vi "Biostinger GUI.vi"() -> ()   [LabVIEW 2014]
uses:
  Controls/State_Enum.ctl
  <vilib>/Utility/file.llb/Write To Spreadsheet File (DBL).vi
panel:
  in  "Clear":bool
  in  "Retraction (um)":dbl
  in  "Penetration (um)":dbl
  out "Waveform Graph":dbl[](graph)
  in  "Zero":bool
  out "XY Graph":cluster{dbl, dbl}[](graph)
  in  "Start Experiment":bool
  in  "Save File":path
  in  "Duration (ms)":u16
  in  "End Voltage (mV)":i16
  in  "Pulse Voltage (mV)":i16
  in  "Current Voltage (mV)":i16
  in  "Command":T1(ring)=enum."Set Statuses"
  in  "Status Value":u16 format="%04x"
  in  "Status Number":u8=61
  in  "Send Command":bool
  out "(hi.lo)":u32[](array[numeric]) format="%8x"
  out "Read Data 4":i32[](array[numeric]) format="%02d"
  in  "Set Parameters":bool
  in  "Start":bool
  in  "Stop":bool
  out "Read Data":u8[](array[numeric]) format="%02x"
  out "Status":string
  out "error out":errorcluster
  in  "error in (no error)":errorcluster
  # "Set Parameters"
  # "Record Data"
  # "Start Experiment"
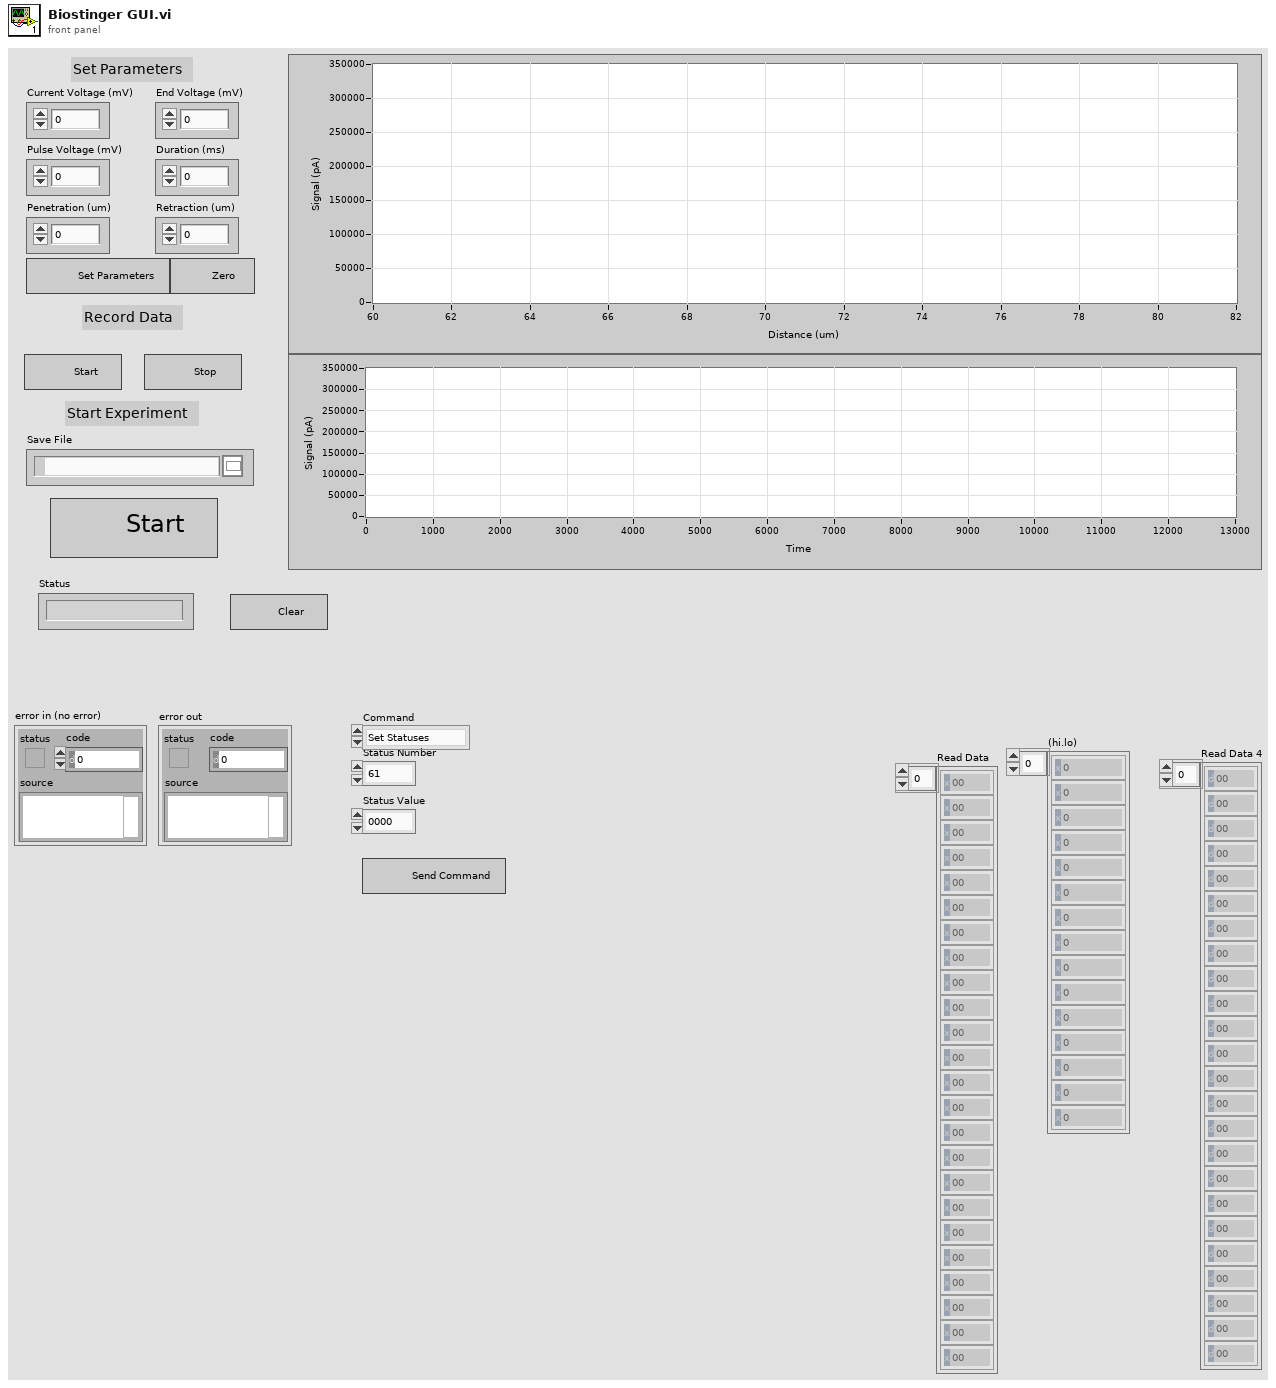
[diagram p1: front panel]
types:
  T1 = enum16{"Default", "Set Statuses", "Set Parameters", "Save Parameter"}
  T2 = typedef "State_Enum.ctl" = enum16{"Init", "Homing", "Homing Done", "Idle", "Zero", "Set Parameters", "Start Collecting Data", "Get Data", "Start Experiment", "Clear Fault", "Send Command", "Stop"}
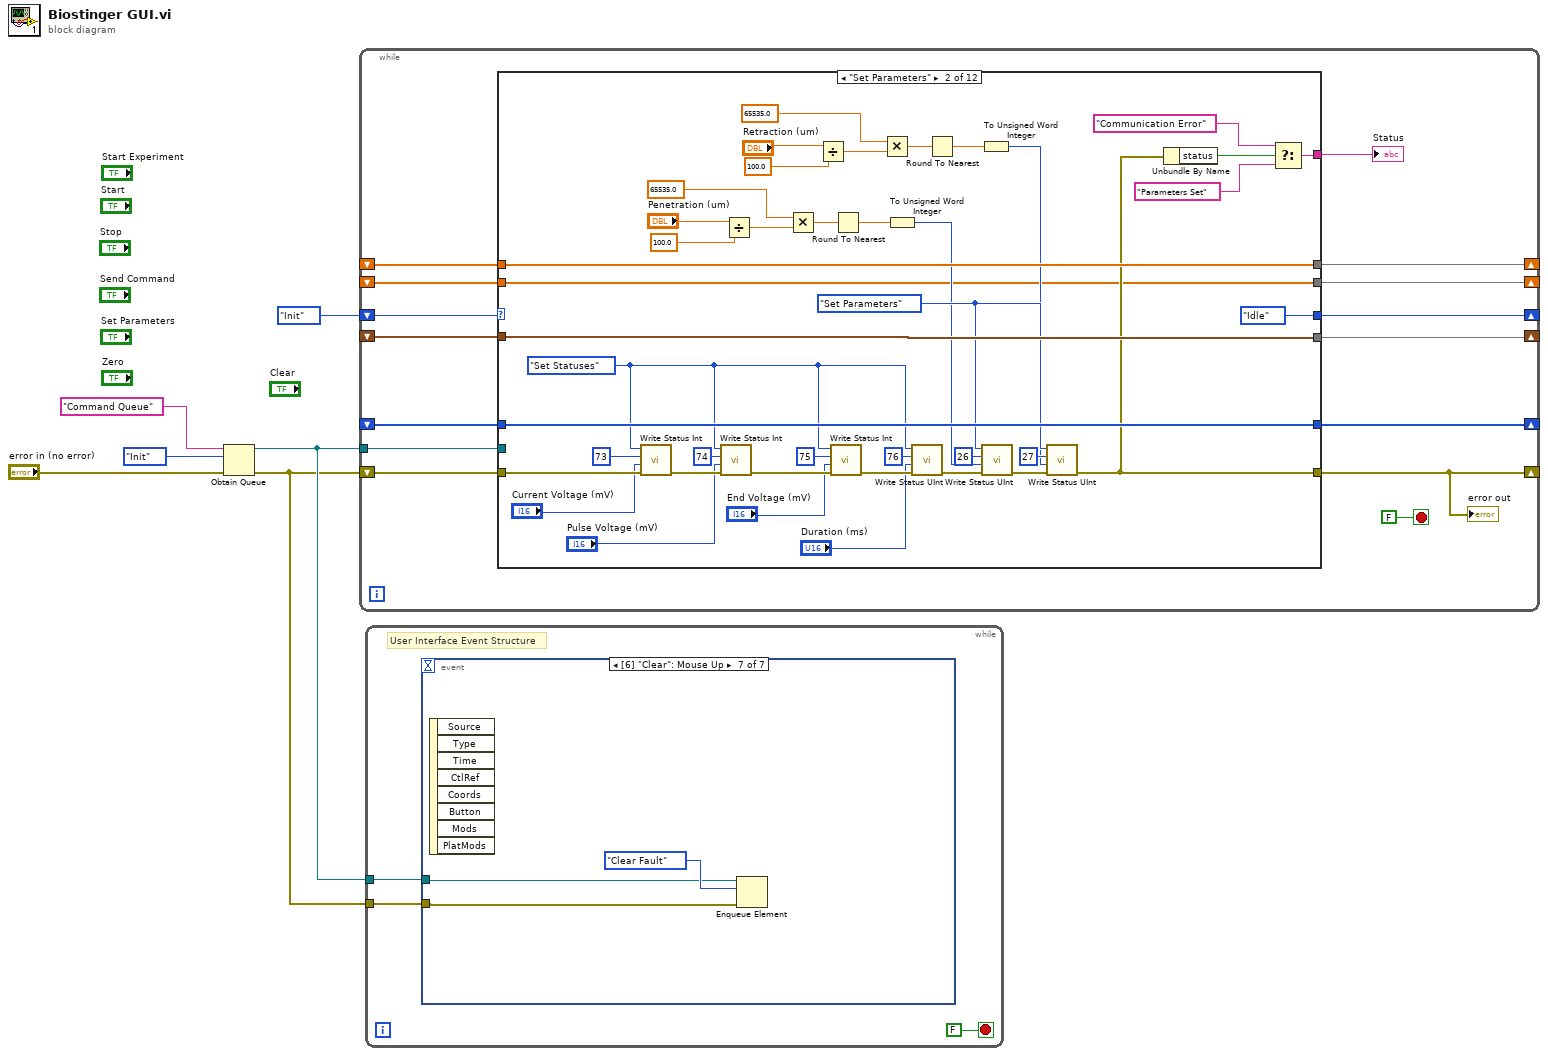
[diagram p0: block diagram]
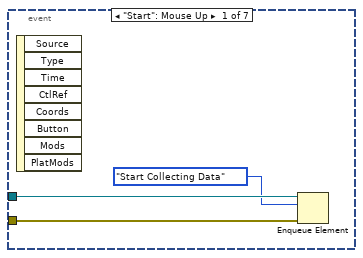
[diagram p2: hidden frame]
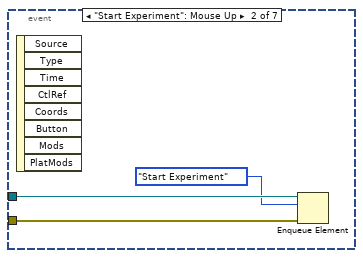
[diagram p3: hidden frame]
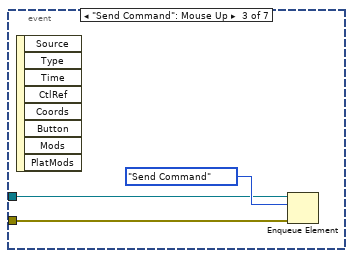
[diagram p4: hidden frame]
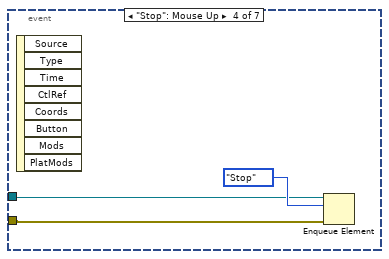
[diagram p5: hidden frame]
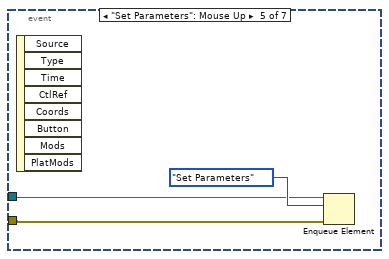
[diagram p6: hidden frame]
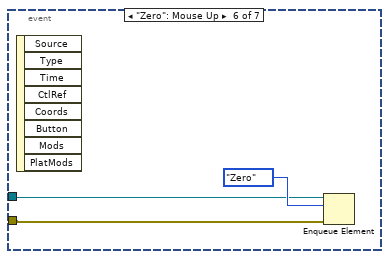
[diagram p7: hidden frame]
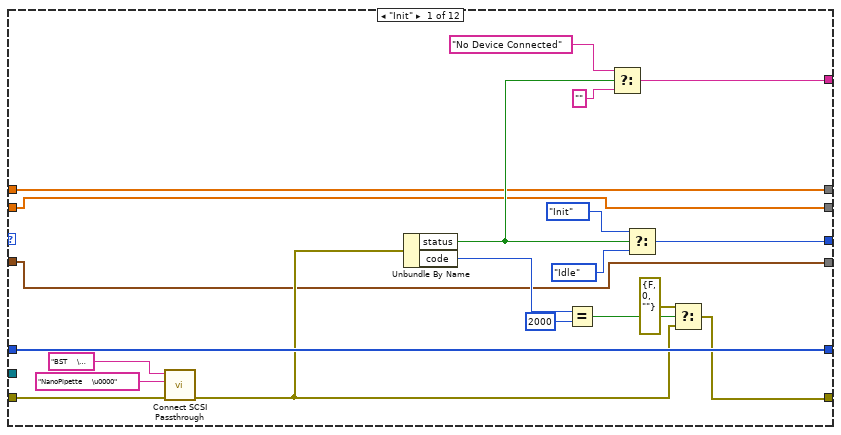
[diagram p8: hidden frame]
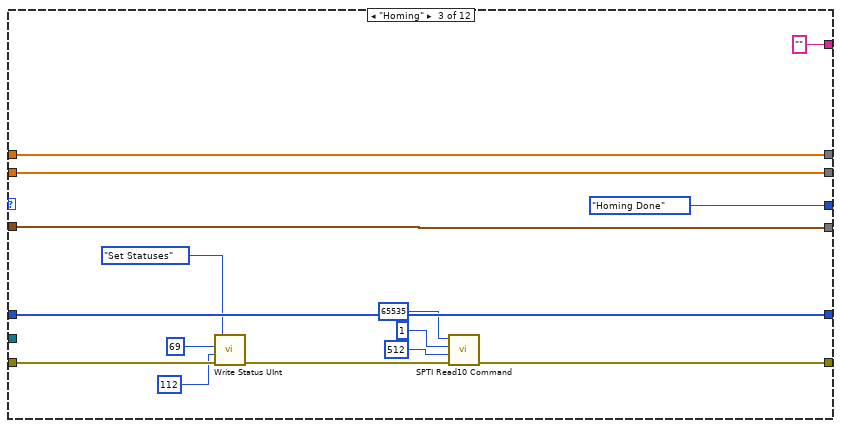
[diagram p9: hidden frame]
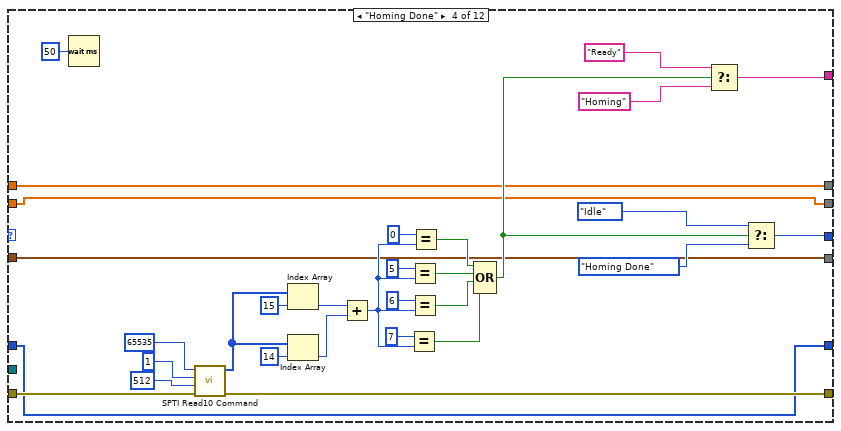
[diagram p10: hidden frame]
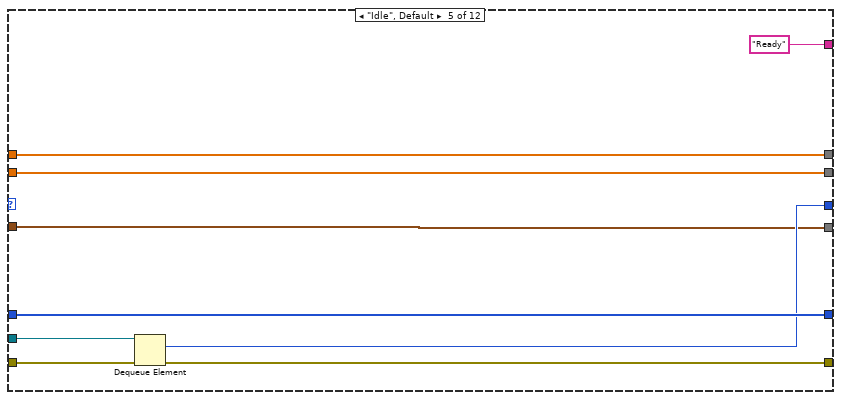
[diagram p11: hidden frame]
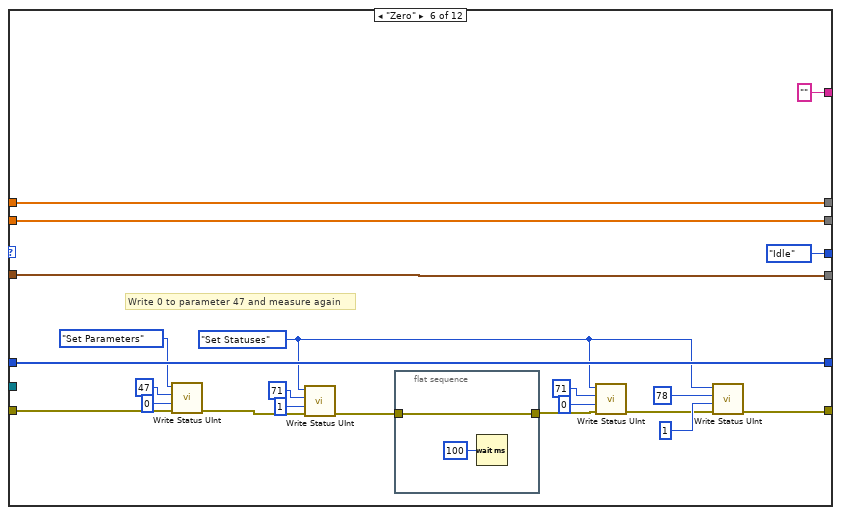
[diagram p12: hidden frame]
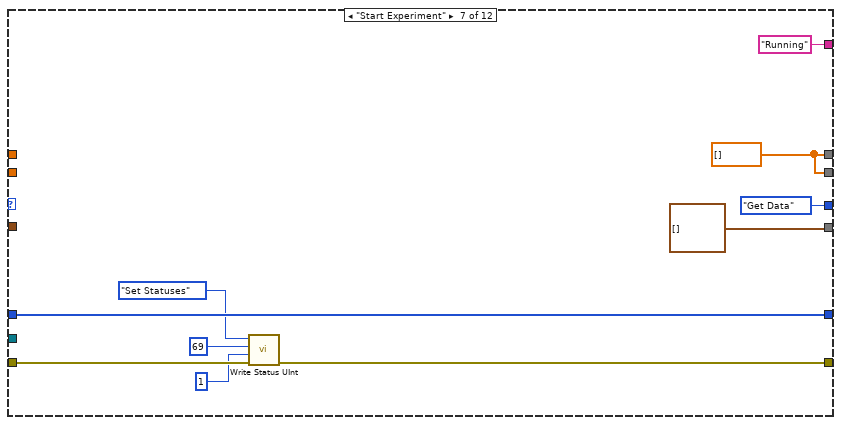
[diagram p13: hidden frame]
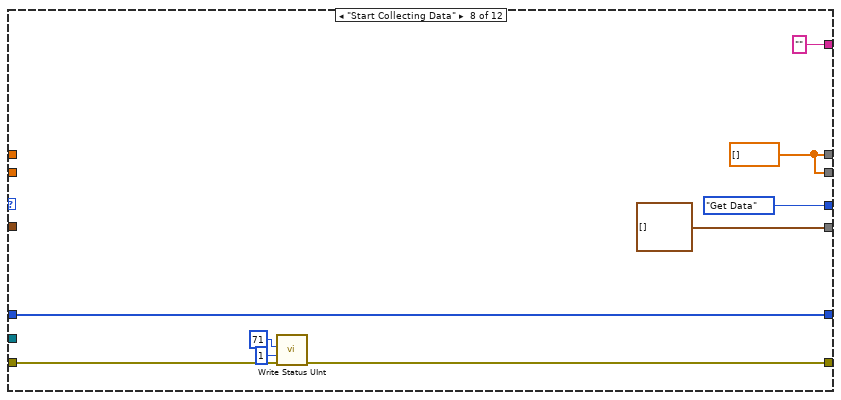
[diagram p14: hidden frame]
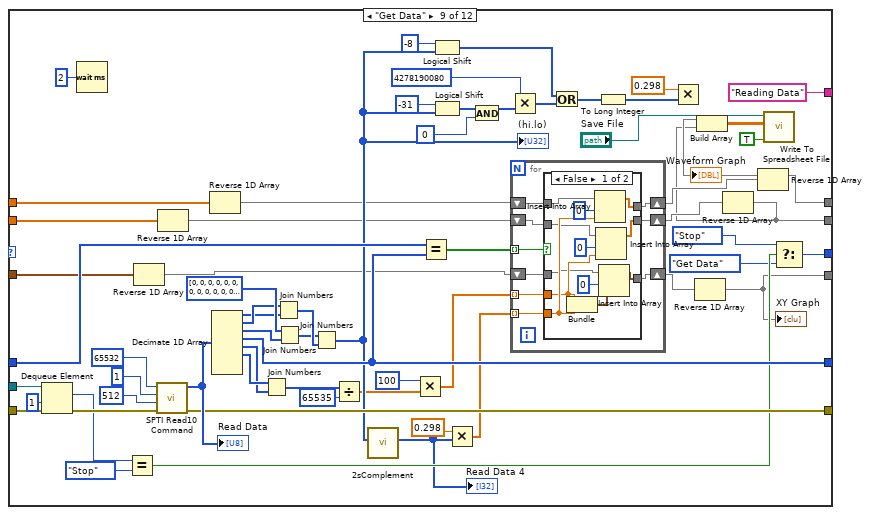
[diagram p15: hidden frame]
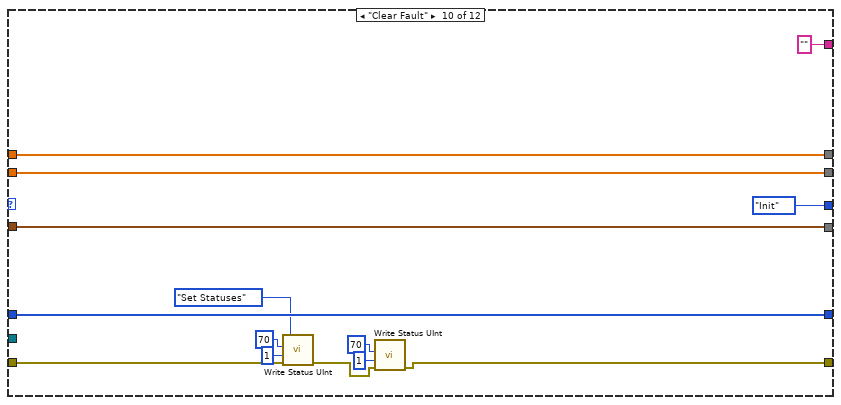
[diagram p17: hidden frame]
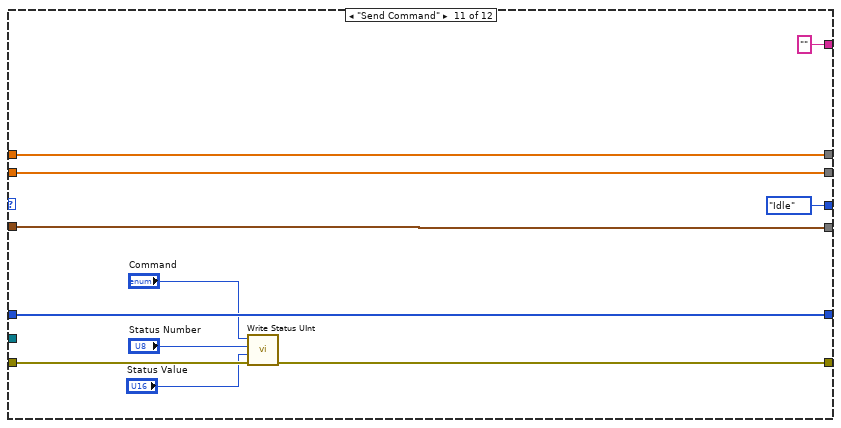
[diagram p18: hidden frame]
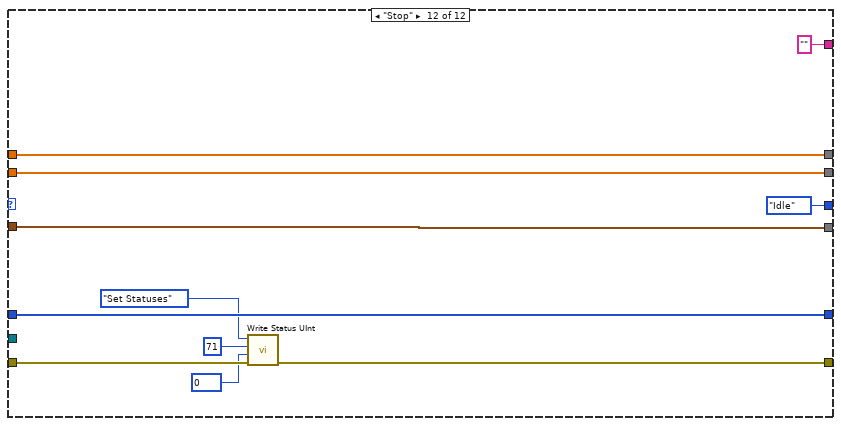
[diagram p19: hidden frame]
diagram:
  n1 = Obtain Queue(name (unnamed)="Command Queue", element data type=State_Enum."Init", error in (no error)="error in (no error)") -> (queue out=w2:refnum<queue>, error out=w1:errorcluster)  [unwired: 2 in, 1 out]
  n2 = while {
    shift-right: [w14] -> _
    shift-left: w1 -> [w20]
    shift-right: [w19] -> _
    shift-left: State_Enum."Init" -> [w21]
    shift-right: [w17] -> _
    shift-left: _ -> [w16]
    tunnel: w2 -> [w15]
    shift-right: [w12] -> _
    shift-left: _ -> [w10]
    shift-right: [w11] -> _
    shift-left: _ -> [w9]
    shift-right: [w8] -> _
    shift-left: _ -> [w7]
    stop <- FALSE stop-if-true
    n3 = case shown="\"Set Parameters\"" w21 {
      tunnel: w20 -> [w39 w82 w96 w124 w135 w140 w169 w178 w214 w273 w289 w300]
      tunnel: [w27 w60 w89 w123 w134 w157 w168 w177 w221 w268 w288 w299] -> w14
      tunnel: [w33 State_Enum."Idle" State_Enum."Homing Done" w127 w132 State_Enum."Idle" State_Enum."Get Data" State_Enum."Get Data" w208 State_Enum."Init" State_Enum."Idle" State_Enum."Idle"] -> w19
      tunnel: [w35 w67 "" ("Status") w102 "Ready" ("Status") "" ("Status") "Running" ("Status") "" ("Status") "Reading Data" ("Status") "" ("Status") "" ("Status") "" ("Status")] -> w18
      tunnel: [w38 w78 w93 w105 w136 w156 w170 w174 w237 w276 w290 w301] -> w17
      tunnel: w16 -> [w38 w78 w93 w105 w136 w156 w170 w174 w234 w276 w290 w301]
      tunnel: w15 -> [_ _ _ _ w133 _ _ _ w213 _ _ _]
      tunnel: [w24 w64 w86 w100 w131 w153 w162 w173 w189 w280 w284 w295] -> w12
      tunnel: [w23 w63 w85 w99 w130 w152 cluster{u16, dbl}[] [] ("XY Graph") cluster{u16, dbl}[] [] ("XY Graph") w181 w278 w283 w294] -> w11
      tunnel: w10 -> [w24 w64 w86 w100 w131 w153 _ _ w192 w280 w284 w295]
      tunnel: w9 -> [w23 w63 w85 w99 w130 w152 _ _ w184 w278 w283 w294]
      tunnel: [w22 w42 w84 w98 w129 w138 w162 w173 w185 w281 w282 w293] -> w8
      tunnel: w7 -> [w22 w42 w84 w98 w129 w138 _ _ w188 w281 w282 w293]
      frame "Init" {
        n4 = call "Connect SCSI Passthrough.vi"("error in (no error)"=w39, "Product"="NanoPipette     \u0000", "Vendor"="BST     \u0000") -> ("error out"=w28:errorcluster)  [unwired: 8 in]
        n5 = Unbundle By Name(w28) -> ("status"=w37:bool, "code"=w29:i32)
        n6 = Equal?(x=w29, y=2000) -> (x = y?=w30:bool)
        n7 = Select(t="No Device Connected", s=w37, f="" ("Status")) -> (s? t:f=w35:string)
        n8 = Select(t=State_Enum."Init", s=w37, f=State_Enum."Idle") -> (s? t:f=w33:T2)
        n9 = Select(t=errorcluster {"status"=FALSE, "code"=0, "source"=""}, s=w30, f=w28) -> (s? t:f=w27:errorcluster)
      }
      frame "Set Parameters" {
        w59 = T1."Set Parameters" ("Command")
        w76 = T1."Set Statuses" ("Command")
        n10 = call "Write Status Int.vi"("error in (no error)"=w82, "Status Value"="Current Voltage (mV)", "Status Number"=u8 73, "Command"=w76) -> ("error out"=w81:errorcluster)  [unwired: 3 in]
        n11 = call "Write Status Int.vi"("error in (no error)"=w81, "Status Value"="Pulse Voltage (mV)", "Status Number"=u8 74, "Command"=w76) -> ("error out"=w80:errorcluster)  [unwired: 3 in]
        n12 = Divide(x="Penetration (um)", y=100.0) -> (x/y=w53:dbl)
        n13 = Multiply(x=65535.0, y=w53) -> (x*y=w51:dbl)
        n14 = Divide(x="Retraction (um)", y=100.0) -> (x/y=w48:dbl)
        n15 = call "Write Status Int.vi"("error in (no error)"=w80, "Status Value"="End Voltage (mV)", "Status Number"=u8 75, "Command"=w76) -> ("error out"=w79:errorcluster)  [unwired: 3 in]
        n16 = Round To Nearest(number=w51) -> (nearest integer value=w50:dbl)
        n17 = Multiply(x=65535.0, y=w48) -> (x*y=w46:dbl)
        n18 = To Unsigned Word Integer(number=w50) -> (unsigned 16bit integer=w56:u16)
        n19 = call "Write Status UInt.vi"("error in (no error)"=w79, "Status Value"="Duration (ms)", "Status Number"=u8 76, "Command"=w76) -> ("error out"=w62:errorcluster)  [unwired: 3 in]
        n20 = Round To Nearest(number=w46) -> (nearest integer value=w45:dbl)
        n21 = To Unsigned Word Integer(number=w45) -> (unsigned 16bit integer=w43:u16)
        n22 = call "Write Status UInt.vi"("error in (no error)"=w62, "Status Value"=w56, "Status Number"=u8 26, "Command"=w59) -> ("error out"=w61:errorcluster)  [unwired: 3 in]
        n23 = call "Write Status UInt.vi"("error in (no error)"=w61, "Status Value"=w43, "Status Number"=u8 27, "Command"=w59) -> ("error out"=w60:errorcluster)  [unwired: 3 in]
        n24 = Unbundle By Name(w60) -> ("status"=w65:bool)
        n25 = Select(t="Communication Error", s=w65, f="Parameters Set" ("Status")) -> (s? t:f=w67:string)
      }
      frame "Homing" {
        n26 = call "Write Status UInt.vi"("error in (no error)"=w96, "Status Value"=u16 112, "Status Number"=u8 69, "Command"=T1."Set Statuses") -> ("error out"=w89:errorcluster)  [unwired: 3 in]
        n27 = call "SPTI Read10 Command.vi"("error in (no error)"=w89, "Block Size (512)"=u32 512, "Nr Blocks"=u32 1, "Start LBA"=u32 65535) -> ()  [unwired: 6 in, 2 out]
      }
      frame "Homing Done" {
        n28 = Wait (ms)(milliseconds to wait=u32 50) -> ()  [unwired: 1 out]
        n29 = call "SPTI Read10 Command.vi"("error in (no error)"=w124, "Block Size (512)"=u32 512, "Nr Blocks"=u32 1, "Start LBA"=u32 65535) -> ("error out"=w123:errorcluster, "Read Data"=w119:u8[])  [unwired: 6 in]
        n30 = Index Array(array=w119, index=15) -> (element=w116:u8)
        n31 = Index Array(array=w119, index=14) -> (element=w115:u8)
        n32 = Add(x=w116, y=w115) -> (x+y=w110:u8)
        n33 = Equal?(x=u8 7, y=w110) -> (x = y?=w106:bool)
        n34 = Equal?(x=u8 5, y=w110) -> (x = y?=w108:bool)
        n35 = Equal?(x=u8 6, y=w110) -> (x = y?=w107:bool)
        n36 = Equal?(x=u8 0, y=w110) -> (x = y?=w109:bool)
        n37 = Compound Arithmetic op=OR(w109, w108, w107, w106) -> (w103:bool)
        n38 = Select(t="Ready", s=w103, f="Homing" ("Status")) -> (s? t:f=w102:string)
        n39 = Select(t=State_Enum."Idle", s=w103, f=State_Enum."Homing Done") -> (s? t:f=w127:T2)
      }
      frame "Idle", Default {
        n40 = Dequeue Element(queue=w133, error in (no error)=w135) -> (element=w132:T2, error out=w134:errorcluster)  [unwired: 1 in, 2 out]
      }
      frame "Zero" {
        w144 = T1."Set Statuses" ("Command")
        # "Write 0 to parameter 47 and measure again"
        n41 = call "Write Status UInt.vi"("error in (no error)"=w140, "Status Value"=u16 0, "Status Number"=u8 47, "Command"=T1."Set Parameters") -> ("error out"=w141:errorcluster)  [unwired: 3 in]
        n42 = call "Write Status UInt.vi"("error in (no error)"=w141, "Status Value"=u16 1, "Status Number"=u8 71, "Command"=w144) -> ("error out"=w146:errorcluster)  [unwired: 3 in]
        n43 = flat-sequence {
          tunnel: w146 -> [w161]
          tunnel: [w161] -> w145
          frame #0 {
            n44 = Wait (ms)(milliseconds to wait=u32 100) -> ()  [unwired: 1 out]
          }
        }
        n45 = call "Write Status UInt.vi"("error in (no error)"=w145, "Status Value"=u16 0, "Status Number"=u8 71, "Command"=w144) -> ("error out"=w147:errorcluster)  [unwired: 3 in]
        n46 = call "Write Status UInt.vi"("error in (no error)"=w147, "Status Value"=u16 1, "Status Number"=u8 78, "Command"=w144) -> ("error out"=w157:errorcluster)  [unwired: 3 in]
      }
      frame "Start Experiment" {
        w162 = dbl[] []
        n47 = call "Write Status UInt.vi"("error in (no error)"=w169, "Status Value"=u16 1, "Status Number"=u8 69, "Command"=T1."Set Statuses") -> ("error out"=w168:errorcluster)  [unwired: 3 in]
      }
      frame "Start Collecting Data" {
        w173 = dbl[] []
        n48 = call "Write Status UInt.vi"("error in (no error)"=w178, "Status Value"=u16 1, "Status Number"=u8 71) -> ("error out"=w177:errorcluster)  [unwired: 4 in]
      }
      frame "Get Data" {
        n49 = Dequeue Element(queue=w213, timeout in ms (-1)=1, error in (no error)=w214) -> (element=w211:T2, error out=w212:errorcluster)  [unwired: 2 out]
        n50 = Wait (ms)(milliseconds to wait=u32 2) -> ()  [unwired: 1 out]
        n51 = Equal?(x=w211, y=State_Enum."Stop") -> (x = y?=w207:bool)
        n52 = Reverse 1D Array(array=w184) -> (reversed array=w183:cluster{dbl, dbl}[])
        n53 = call "SPTI Read10 Command.vi"("error in (no error)"=w212, "Block Size (512)"=u32 512, "Nr Blocks"=u32 1, "Start LBA"=u32 65532) -> ("error out"=w221:errorcluster, "Read Data"=w238:u8[])  [unwired: 6 in]
        "Read Data" <- w238
        n54 = Reverse 1D Array(array=w188) -> (reversed array=w187:dbl[])
        n55 = Reverse 1D Array(array=w192) -> (reversed array=w191:dbl[])
        n56 = Decimate 1D Array(w238) -> (w217:u8[], w218:u8[], w219:u8[], w237:u8[], w203:u8[], w204:u8[])  [unwired: 2 out]
        n57 = Join Numbers(hi=w204, lo=w203) -> ((hi.lo)=w200:u16[])
        n58 = Join Numbers(hi=w218, lo=w217) -> ((hi.lo)=w236:u16[])
        n59 = Join Numbers(hi=u8[] [0, 0, 0, 0, 0, 0, 0, 0, 0, 0, 0, 0, 0, 0, 0, 0, 0, 0, 0, 0, 0, 0, 0, 0, 0, 0, 0, 0, 0, 0, 0, 0] ("decimated array"), lo=w219) -> ((hi.lo)=w231:u16[])
        n60 = Join Numbers(hi=w231, lo=w236) -> ((hi.lo)=w202:u32[])
        "(hi.lo)" <- w202
        n61 = Divide(x=w200, y=65535) -> (x/y=w198:dbl[])
        n62 = call "2sComplement.vi"("Data In"=w202) -> ("Data Out"=w201:i32[])  [unwired: 10 in]
        "Read Data 4" <- w201
        n63 = Multiply(x=100, y=w198) -> (x*y=w196:dbl[])
        n64 = Equal?(x=w234, y=w237) -> (x = y?=w216:bool[])
        n65 = Logical Shift(y=i16 -8, x=w202) -> (x << y=w223:u32[])
        n66 = Logical Shift(y=i16 -31, x=w202) -> (x << y=w228:u32[])
        n67 = Multiply(x=0.298, y=w201) -> (x*y=w215:dbl[])
        n68 = And(x=w228, y=u32 0) -> (x .and. y?=w226:u32[])
        n69 = Multiply(x=u32 4278190080, y=w226) -> (x*y=w224:u32[])
        n70 = for {
          tunnel: w216 -> [w252] mode=indexing
          tunnel: w215 -> [w250] mode=indexing
          shift-right: [w249] -> w182
          shift-left: w183 -> [w251]
          tunnel: w196 -> [w248] mode=indexing
          shift-right: [w247] -> w190
          shift-left: w191 -> [w246]
          shift-right: [w245] -> w186
          shift-left: w187 -> [w244]
          n71 = case shown="False" w252 {
            tunnel: w251 -> [w254 w266]
            tunnel: w250 -> [w263 _]
            tunnel: [w253 w266] -> w249
            tunnel: w248 -> [w259 _]
            tunnel: [w261 w267] -> w247
            tunnel: w246 -> [w264 w267]
            tunnel: [w257 w265] -> w245
            tunnel: w244 -> [w258 w265]
            frame False {
              n72 = Bundle(w259, w263) -> (w255:cluster{dbl, dbl})  [unwired: 1 in]
              n73 = Insert Into Array(array=w264, index=0, new element=w263) -> (w261:dbl[])
              n74 = Insert Into Array(array=w258, index=0, new element=w259) -> (w257:dbl[])
              n75 = Insert Into Array(array=w254, index=0, new element=w255) -> (w253:cluster{dbl, dbl}[])
            }
            frame True {
            }
          }
        }
        n76 = Or(x=w223, y=w224) -> (x .or. y?=w222:u32[])
        n77 = To Long Integer(number=w222) -> (32bit integer=w232:i32[])
        n78 = Multiply(x=0.298, y=w232) -> ()  [unwired: 1 out]
        n79 = Reverse 1D Array(array=w182) -> (reversed array=w181:cluster{dbl, dbl}[])
        "XY Graph" <- w181
        n80 = Reverse 1D Array(array=w186) -> (reversed array=w185:dbl[])
        n81 = Reverse 1D Array(array=w190) -> (reversed array=w189:dbl[])
        "Waveform Graph" <- w189
        n82 = Build Array(w189, w185) -> (w193:dbl[][])
        n83 = call-poly <vilib>:"Write To Spreadsheet File.vi"("append to file? (new file:F)"=TRUE, "2D data"=w193, "file path (dialog if empty)"="Save File") -> ()  [unwired: 5 in, 1 out]
        n84 = Select(t=State_Enum."Stop", s=w207, f=State_Enum."Get Data") -> (s? t:f=w208:T2)
      }
      frame "Clear Fault" {
        n85 = call "Write Status UInt.vi"("error in (no error)"=w273, "Status Value"=u16 1, "Status Number"=u8 70, "Command"=T1."Set Statuses") -> ("error out"=w269:errorcluster)  [unwired: 3 in]
        n86 = call "Write Status UInt.vi"("error in (no error)"=w269, "Status Value"=u16 1, "Status Number"=u8 70) -> ("error out"=w268:errorcluster)  [unwired: 4 in]
      }
      frame "Send Command" {
        n87 = call "Write Status UInt.vi"("error in (no error)"=w289, "Status Value"="Status Value", "Status Number"="Status Number", "Command"="Command") -> ("error out"=w288:errorcluster)  [unwired: 3 in]
      }
      frame "Stop" {
        n88 = call "Write Status UInt.vi"("error in (no error)"=w300, "Status Value"=u16 0 ("Status Value 2"), "Status Number"=u8 71 ("Status Number 2"), "Command"=T1."Set Statuses" ("Command 2")) -> ("error out"=w299:errorcluster)  [unwired: 3 in]
      }
    }
    "Status" <- w18
    "error out" <- w14
  }
  n89 = while {
    tunnel: w2 -> [w306]
    tunnel: w1 -> [w305]
    stop <- FALSE stop-if-true
    # "User Interface Event Structure"
    n90 = event shown="[6] \"Clear\": Mouse Up" {
      selector: _ -> [_ _ _ _ _ _ _]
      dyn-events: _ -> [_ _ _ _ _ _ _]
      timeout: _ -> [_ _ _ _ _ _ _]
      tunnel: w306 -> [w309 w312 w314 w317 w320 w323 w326]
      tunnel: w305 -> [w308 w311 w313 w316 w319 w322 w325]
      event "Start": Mouse Up {
        n91 = event-data() -> ()  [unwired: 1 in, 8 out]
        n92 = Enqueue Element(queue=w309, element=State_Enum."Start Collecting Data", error in (no error)=w308) -> ()  [unwired: 1 in, 3 out]
      }
      event "Start Experiment": Mouse Up {
        n93 = event-data() -> ()  [unwired: 1 in, 8 out]
        n94 = Enqueue Element(queue=w312, element=State_Enum."Start Experiment", error in (no error)=w311) -> ()  [unwired: 1 in, 3 out]
      }
      event "Send Command": Mouse Up {
        n95 = event-data() -> ()  [unwired: 1 in, 8 out]
        n96 = Enqueue Element(queue=w314, element=State_Enum."Send Command", error in (no error)=w313) -> ()  [unwired: 1 in, 3 out]
      }
      event "Stop": Mouse Up {
        n97 = event-data() -> ()  [unwired: 1 in, 8 out]
        n98 = Enqueue Element(queue=w317, element=State_Enum."Stop", error in (no error)=w316) -> ()  [unwired: 1 in, 3 out]
      }
      event "Set Parameters": Mouse Up {
        n99 = event-data() -> ()  [unwired: 1 in, 8 out]
        n100 = Enqueue Element(queue=w320, element=State_Enum."Set Parameters", error in (no error)=w319) -> ()  [unwired: 1 in, 3 out]
      }
      event "Zero": Mouse Up {
        n101 = event-data() -> ()  [unwired: 1 in, 8 out]
        n102 = Enqueue Element(queue=w323, element=State_Enum."Zero", error in (no error)=w322) -> ()  [unwired: 1 in, 3 out]
      }
      event "Clear": Mouse Up {
        n103 = event-data() -> ()  [unwired: 1 in, 8 out]
        n104 = Enqueue Element(queue=w326, element=State_Enum."Clear Fault", error in (no error)=w325) -> ()  [unwired: 1 in, 3 out]
      }
    }
  }
